vi "ZCR Find state by thresholds.vi"(10 "Noise amplitude":dbl format="%.2p", 11 "ZCR IN":waveform(dbl)[](array[waveform])=[{"t0"=timestamp(3707890383.8976955 s since 1904-01-01), "dt"=9.999999999999999e-05, "Y"=array[20000 elements], "attributes"=variant("NI_ChannelName"=variant(string "Tension_0"), "NI_UnitDescription"=variant(string "Volts"))}, {"t0"=timestamp(3707890383.8977456 s since 1904-01-01), "dt"=9.999999999999999e-05, "Y"=array[20000 elements], "attributes"=variant("NI_ChannelName"=variant(string "Tension_1"), "NI_UnitDescription"=variant(string "Volts"))}]) -> (2 "SIN OFF Points":i32[](array[numeric]), 3 "SIN ON Points":i32[](array[numeric]))   [LabVIEW 2020, in "Library Commun.lvlib" / "Nodon_ZCR.lvclass"]
uses:
  Nodon_ZCR.lvclass
  <vilib>/Utility/miscctls.llb/LVRangeTypeDef.ctl
  Nodon_ZCR.lvclass/Nodon_ZCR.ctl
  <vilib>/measure/NI_MABase.lvlib
panel:
  in  "Point for zoom":i32
  out "Input Signal":waveform(dbl)[](graph)
  # "This VI Find the ON states and the OFF states based on a fix value\nNot to be used of ZCR control, due to the thresholds noise close to 0"
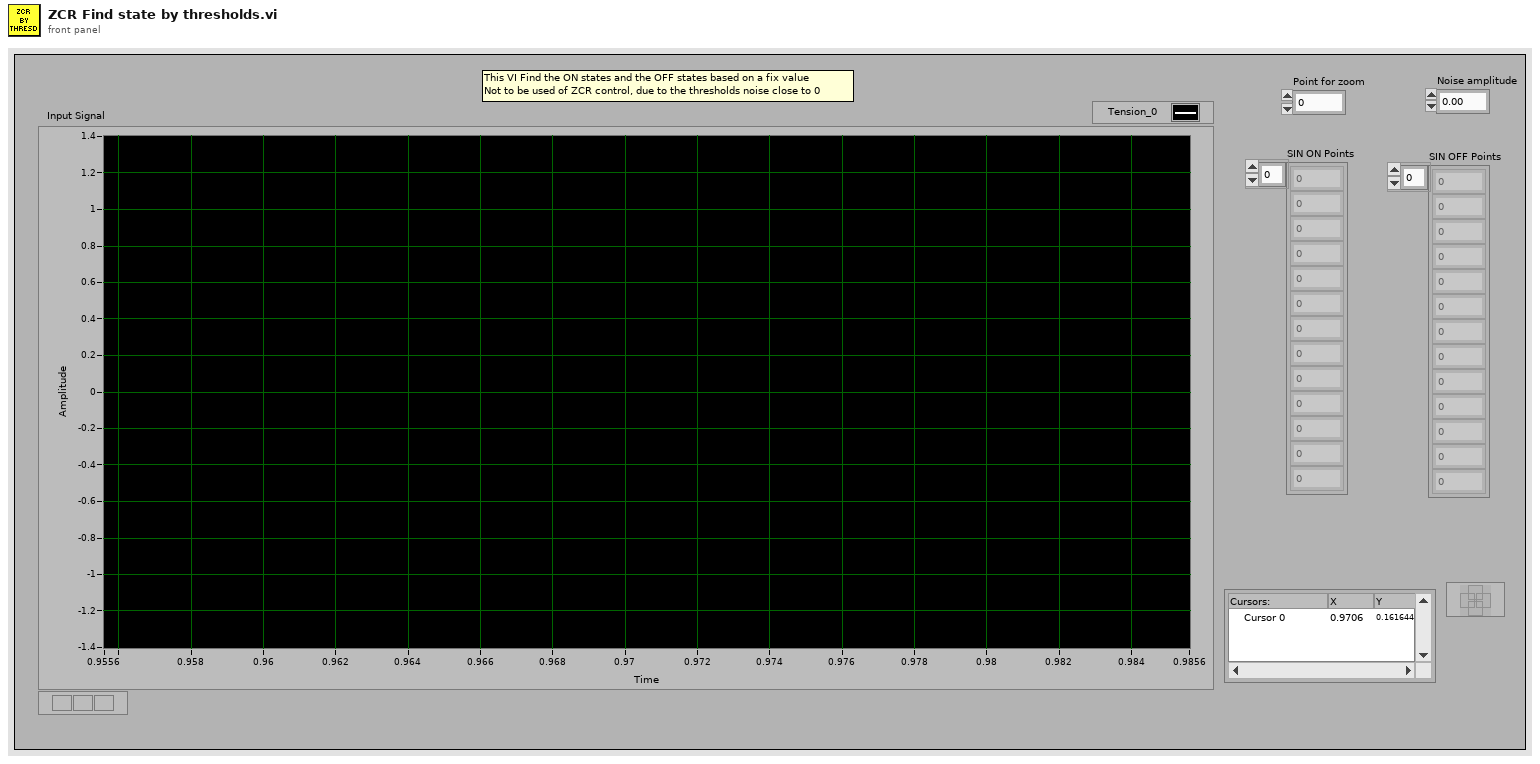
[diagram p1: front panel]
types:
  T1 = typedef "LVRangeTypeDef.ctl" = cluster{"Minimum":dbl, "Maximum":dbl, "Increment":dbl, "Minor Increment":dbl, "Start":dbl}
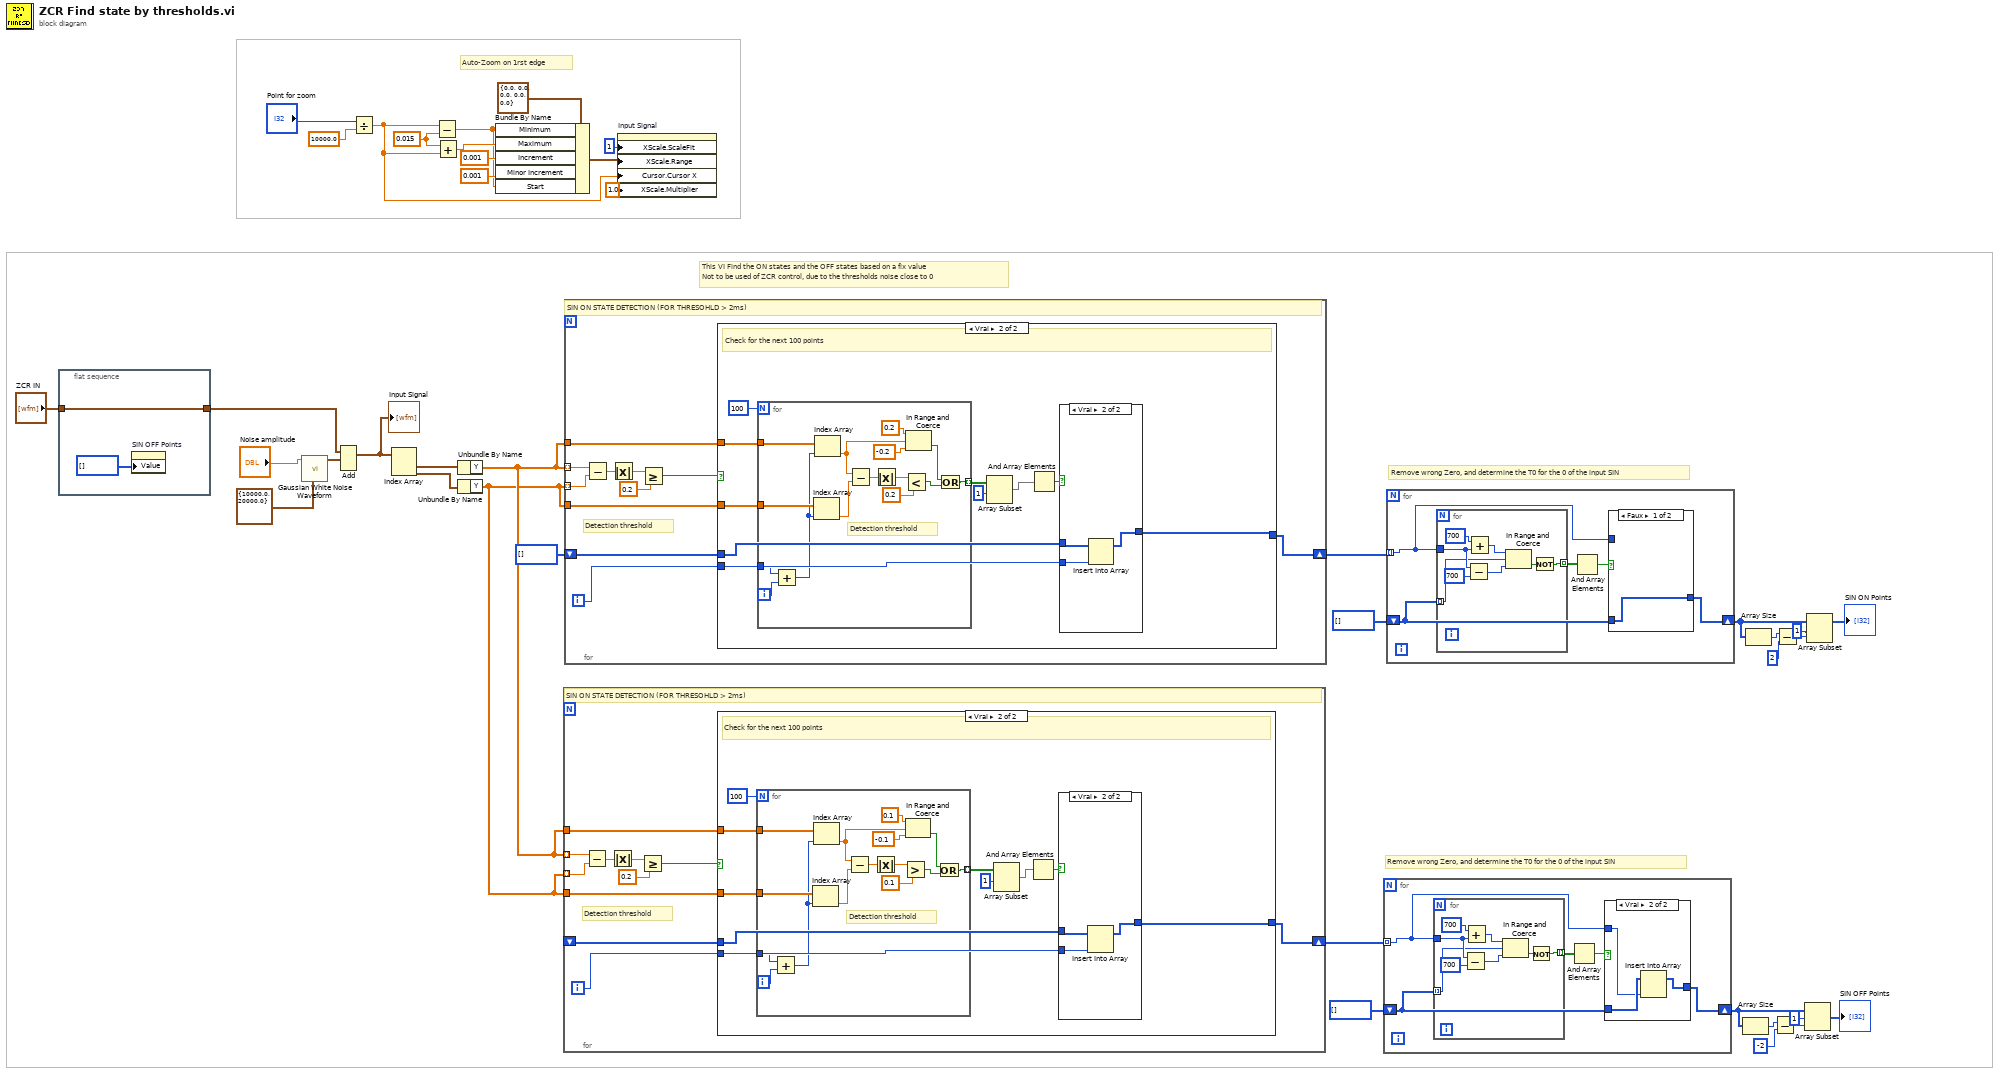
[diagram p0: block diagram]
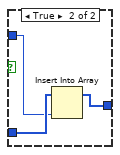
[diagram p2: hidden frame]
diagram:
  w32 = 0.015
  # "Remove wrong Zero, and determine the T0 for the 0 of the input SIN"
  # "Remove wrong Zero, and determine the T0 for the 0 of the input SIN"
  # "This VI Find the ON states and the OFF states based on a fix value\nNot to be used of ZCR control, due to the thresholds noise close to 0"
  # "Auto-Zoom on 1rst edge"
  n1 = flat-sequence {
    tunnel: "ZCR IN" -> [w40]
    tunnel: [w40] -> w2
    frame #0 {
      n2 = property on="SIN OFF Points" class="Tabl (strict)"("Value"=i32[] []) -> ()  [unwired: 2 in, 2 out]
    }
  }
  n3 = call <vilib>:"Gaussian White Noise Waveform.vi"("sampling info"=cluster{"Fs":dbl, "#s":dbl} {"Fs"=10000.0, "#s"=20000.0}, "standard deviation"="Noise amplitude") -> ("signal out"=w38:waveform(dbl))  [unwired: 8 in, 1 out]
  n4 = Add(1:w38, 2:w2) -> (0:w37:waveform(dbl)[])  [unwired: 1 in, 1 out]
  "Input Signal" <- w37
  n5 = Divide(x="Point for zoom", y=10000.0) -> (x/y=w23:dbl)
  n6 = Index Array(array=w37) -> (element #1=w36:waveform(dbl), element #2=w35:waveform(dbl))  [unwired: 2 in]
  n7 = Subtract(x=w23, y=w32) -> (x-y=w27:dbl)
  n8 = Add(x=w32, y=w23) -> (x+y=w30:dbl)
  n9 = Unbundle By Name(w36) -> ("Y"=w22:dbl[])
  n10 = Unbundle By Name(w35) -> ("Y"=w1:dbl[])
  n11 = Bundle By Name(cluster=T1 {"Minimum"=0.0, "Maximum"=0.0, "Increment"=0.0, "Minor Increment"=0.0, "Start"=0.0} ("X Scale.Range"), "Minimum"=w27, "Maximum"=w30, "Increment"=0.001, "Minor Increment"=0.001, "Start"=w27) -> (w26:T1)
  n12 = for {
    tunnel: w22 -> [w52] mode=indexing
    tunnel: w1 -> [w51] mode=indexing
    shift-right: [w44] -> w20
    shift-left: _ -> [w46]
    tunnel: w1 -> [w43]
    tunnel: w22 -> [w42]
    i -> [w45]
    # "Detection threshold"
    # "SIN ON STATE DETECTION (FOR THRESOHLD > 2ms)"
    n13 = Subtract(x=w52, y=w51) -> (x-y=w50:dbl)
    n14 = Absolute Value(x=w50) -> (abs(x)=w49:dbl)
    n15 = Greater Or Equal?(x=w49, y=0.2) -> (x >= y?=w47:bool)
    n16 = case shown="Vrai" w47 {
      tunnel: w46 -> [w53 w59]
      tunnel: w45 -> [_ w58]
      tunnel: [w53 w57] -> w44
      tunnel: w43 -> [_ w61]
      tunnel: w42 -> [_ w62]
      frame False {
      }
      frame True {
        # "Check for the next 100 points"
        n17 = for {
          N: 100 -> [_]
          tunnel: w62 -> [w82]
          tunnel: w61 -> [w80]
          tunnel: w58 -> [w74]
          tunnel: [w68] -> w56 mode=indexing
          i -> [w81]
          # "Detection threshold"
          n18 = Add(x=w74, y=w81) -> (x+y=w79:i32)
          n19 = Index Array(array=w80, index=w79) -> (element=w75:dbl)
          n20 = Index Array(array=w82, index=w79) -> (element=w73:dbl)
          n21 = Subtract(x=w73, y=w75) -> (x-y=w78:dbl)
          n22 = Absolute Value(x=w78) -> (abs(x)=w77:dbl)
          n23 = Greater?(x=w77, y=0.1) -> (0:w70:bool)
          n24 = In Range and Coerce(upper limit=0.1, x=w73, lower limit=-0.1) -> (In Range?=w69:bool)  [unwired: 1 out]
          n25 = Or(x=w69, y=w70) -> (x .or. y?=w68:bool)
        }
        n26 = Array Subset(array=w56, index=1) -> (w55:bool[])  [unwired: 1 in]
        n27 = And Array Elements(Boolean array=w55) -> (logical AND=w60:bool)
        n28 = case shown="Vrai" w60 {
          tunnel: w59 -> [w64 w66]
          tunnel: w58 -> [_ w67]
          tunnel: [w64 w65] -> w57
          frame False {
          }
          frame True {
            n29 = Insert Into Array(array=w66, new element=w67) -> (w65:i32[])  [unwired: 1 in]
          }
        }
      }
    }
  }
  n30 = for {
    tunnel: w22 -> [w93] mode=indexing
    tunnel: w1 -> [w92] mode=indexing
    shift-right: [w85] -> w18
    shift-left: i32[] [] -> [w87]
    tunnel: w1 -> [w84]
    tunnel: w22 -> [w83]
    i -> [w86]
    # "Detection threshold"
    # "SIN ON STATE DETECTION (FOR THRESOHLD > 2ms)"
    n31 = Subtract(x=w93, y=w92) -> (x-y=w91:dbl)
    n32 = Absolute Value(x=w91) -> (abs(x)=w90:dbl)
    n33 = Greater Or Equal?(x=w90, y=0.2) -> (x >= y?=w88:bool)
    n34 = case shown="Vrai" w88 {
      tunnel: w87 -> [w94 w100]
      tunnel: w86 -> [_ w99]
      tunnel: [w94 w98] -> w85
      tunnel: w84 -> [_ w102]
      tunnel: w83 -> [_ w103]
      frame False {
      }
      frame True {
        # "Check for the next 100 points"
        n35 = for {
          N: 100 -> [_]
          tunnel: w103 -> [w123]
          tunnel: w102 -> [w121]
          tunnel: w99 -> [w115]
          tunnel: [w109] -> w97 mode=indexing
          i -> [w122]
          # "Detection threshold"
          n36 = Add(x=w115, y=w122) -> (x+y=w120:i32)
          n37 = Index Array(array=w121, index=w120) -> (element=w116:dbl)
          n38 = Index Array(array=w123, index=w120) -> (element=w114:dbl)
          n39 = Subtract(x=w114, y=w116) -> (x-y=w119:dbl)
          n40 = Absolute Value(x=w119) -> (abs(x)=w118:dbl)
          n41 = Less?(x=w118, y=0.2) -> (x < y?=w111:bool)
          n42 = In Range and Coerce(upper limit=0.2, x=w114, lower limit=-0.2) -> (In Range?=w110:bool)  [unwired: 1 out]
          n43 = Or(x=w110, y=w111) -> (x .or. y?=w109:bool)
        }
        n44 = Array Subset(array=w97, index=1) -> (w96:bool[])  [unwired: 1 in]
        n45 = And Array Elements(Boolean array=w96) -> (logical AND=w101:bool)
        n46 = case shown="Vrai" w101 {
          tunnel: w100 -> [w105 w107]
          tunnel: w99 -> [_ w108]
          tunnel: [w105 w106] -> w98
          frame False {
          }
          frame True {
            n47 = Insert Into Array(array=w107, new element=w108) -> (w106:i32[])  [unwired: 1 in]
          }
        }
      }
    }
  }
  n48 = property on="Input Signal" class="GraphWF (strict)"("XScale.ScaleFit"=u8 1 ("X Scale.Scale Fit"), "XScale.Range"=w26, "Cursor.Cursor X"=w23, "XScale.Multiplier"=1.0 ("X Scale.Offset and Multiplier:Multiplier")) -> ()  [unwired: 2 in, 2 out]
  n49 = for {
    tunnel: w20 -> [w126] mode=indexing
    shift-right: [w127] -> w11
    shift-left: i32[] [] -> [w128]
    n50 = for {
      tunnel: w126 -> [w136]
      tunnel: w128 -> [w133] mode=indexing
      tunnel: [w134] -> w125 mode=indexing
      n51 = Subtract(x=w136, y=700) -> (x-y=w137:i32)
      n52 = Add(x=700, y=w136) -> (x+y=w138:i32)
      n53 = In Range and Coerce(upper limit=w138, x=w133, lower limit=w137) -> (In Range?=w135:bool)  [unwired: 1 out]
      n54 = Not(x=w135) -> (.not. x?=w134:bool)
    }
    n55 = And Array Elements(Boolean array=w125) -> (logical AND=w124:bool)
    n56 = case shown="Vrai" w124 {
      tunnel: w128 -> [w129 w131]
      tunnel: [w129 w132] -> w127
      tunnel: w126 -> [_ w130]
      frame False {
      }
      frame True {
        n57 = Insert Into Array(array=w131, new element=w130) -> (w132:i32[])  [unwired: 1 in]
      }
    }
  }
  n58 = for {
    tunnel: w18 -> [w143] mode=indexing
    shift-right: [w144] -> w14
    shift-left: i32[] [] -> [w145]
    n59 = for {
      tunnel: w143 -> [w153]
      tunnel: w145 -> [w150] mode=indexing
      tunnel: [w151] -> w142 mode=indexing
      n60 = Subtract(x=w153, y=700) -> (x-y=w154:i32)
      n61 = Add(x=700, y=w153) -> (x+y=w155:i32)
      n62 = In Range and Coerce(upper limit=w155, x=w150, lower limit=w154) -> (In Range?=w152:bool)  [unwired: 1 out]
      n63 = Not(x=w152) -> (.not. x?=w151:bool)
    }
    n64 = And Array Elements(Boolean array=w142) -> (logical AND=w141:bool)
    n65 = case shown="Faux" w141 {
      tunnel: w145 -> [w146 w148]
      tunnel: [w146 w149] -> w144
      tunnel: w143 -> [_ w147]
      frame False {
      }
      frame True {
        n66 = Insert Into Array(array=w148, new element=w147) -> (w149:i32[])  [unwired: 1 in]
      }
    }
  }
  n67 = Array Size(array=w11) -> (size(s)=w5:i32)
  n68 = Array Size(array=w14) -> (size(s)=w7:i32)
  n69 = Subtract(x=w5, y=-2) -> (x-y=w12:i32)
  n70 = Subtract(x=w7, y=2) -> (x-y=w13:i32)
  n71 = Array Subset(array=w11, index=1, length=w12) -> (→"SIN OFF Points":i32[])
  n72 = Array Subset(array=w14, index=1, length=w13) -> (→"SIN ON Points":i32[])
